vi "ClientFinalNoProof.vi"(8 "error in (no error)":errorcluster, 10 "Authenticate Extra  Data":T1, 11 "WampScramAuthenticator in":refnum<class "WampScramAuthenticator.lvclass">) -> (0 "error out":errorcluster, 1 "ClientFinalNoProof":string, 2 "Authenticate Extra  Data":T1, 3 "WampScramAuthenticator out":refnum<class "WampScramAuthenticator.lvclass">)   [LabVIEW 2020, in "wamplv.lvlib" / "WampScramAuthenticator.lvclass"]
uses:
  WampScramAuthenticator.lvclass
  TypeDefs/Authenticate Extra data.ctl
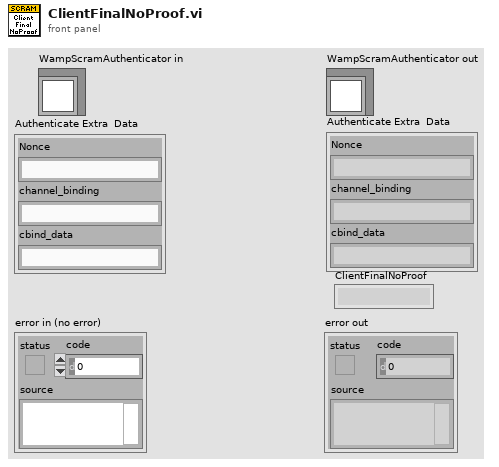
[diagram p1: front panel]
types:
  T1 = typedef "wamplv.lvlib/WampScramAuthenticator.lvclass/Authenticate Extra data.ctl" = cluster{"Nonce":string, "channel_binding":string, "cbind_data":string}
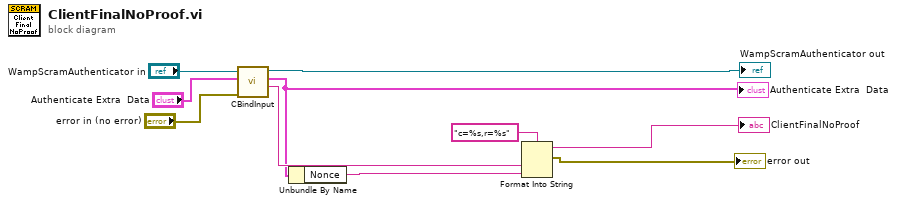
[diagram p0: block diagram]
diagram:
  n1 = call "CBindInput.vi"("error in (no error)"="error in (no error)", "Authenticate Extra  Data"="Authenticate Extra  Data", "WampScramAuthenticator in"="WampScramAuthenticator in") -> ("CBindInput"=w4:string, "Authenticate Extra Data"=w2:T1, "WampScramAuthenticator out"=→"WampScramAuthenticator out":refnum<class "WampScramAuthenticator.lvclass">)  [unwired: 5 in, 1 out]
  "Authenticate Extra  Data" <- w2
  n2 = Unbundle By Name(w2) -> ("Nonce"=w3:string)
  n3 = Format Into String(format string="c=%s,r=%s", w4, w3) -> (resulting string=→"ClientFinalNoProof":string, error out=→"error out":errorcluster)  [unwired: 2 in]
